vi "BGK Data Acquisition Loop - FCXF.vi"(7 "Period (s)":dbl=600.0 caption="采样周期 (s)" format="%#_13g", 8 "error in (no error)":errorcluster caption="错误输入（无错误）", 11 "Message Queues":T1 caption="消息队列") -> (0 "error out":errorcluster caption="错误输出")   [LabVIEW 2015]
uses:
  Support VIs/Message Queue/All Real-Time Message Queues.ctl
  Support VIs/Message Queue/Message Cluster.ctl
  <vilib>/Platform/TimedLoop/XDataNode/timing_clust.ctl
  <vilib>/Platform/TimedLoop/XDataNode/nitl_modes.ctl
  <vilib>/Platform/TimedLoop/XDataNode/wakeup.ctl
  <vilib>/Instr/_visa.llb/VISA Configure Serial Port (Instr).vi
  Globals/Global - Monitoring Variables.vi
  <vilib>/Platform/TimedLoop/XDataNode/loadnilvce.vi
  Globals/Global - All RT Loop Stop.vi
  <vilib>/Platform/TimedLoop/XDataNode/XDataNode.xnode
  <vilib>/Platform/TimedLoop/XDataNode/XDNodeRunTimeDep.lvlib
  Support VIs/Message Queue/Message Queue.lvlib
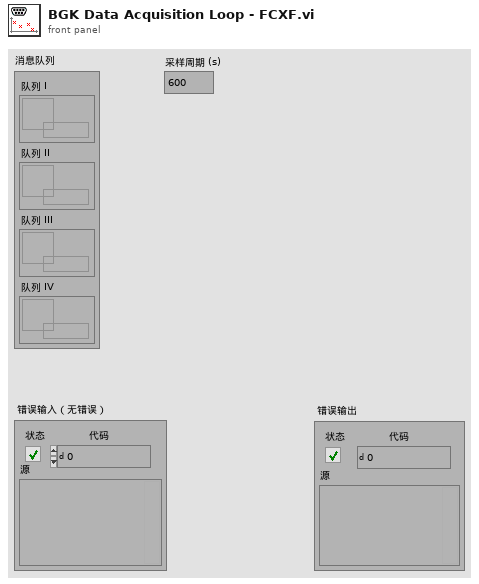
[diagram p1: front panel]
types:
  T1 = typedef "Message Queue.lvlib/All Real-Time Message Queues.ctl" = cluster{"Queue I":refnum<queue>, "Queue II":refnum<queue>, "Queue III":refnum<queue>, "Queue IV":refnum<queue>}
  T2 = typedef "XDNodeRunTimeDep.lvlib/timing_clust.ctl" = cluster{"Expected End [f-1]":u64, "Actual End [f-1]":u64, "Finished Late? [f-1]":bool, "Expected End [i-1]":u64, "Actual End [i-1]":u64, "Finished Late? [i-1]":bool, "Expected Start [i]":u64, "Actual Start [i]":u64, "Expected Start [f]":u64, "Actual Start [f]":u64, "Source Name":string, "Structure Name":string, "Period":i64, "Deadline":i64, "Offset":i64, "Start":i64, "Priority":i32, "Timeout":i32, "Mode":T3, "Wakeup Reason":T4, "Error":errorcluster, "Source Type":string, "Secondary Source Type":string, "Global End Time":u64, "Global Start Time":u64, "Frame Duration":u64, "Iteration Duration":u64, "Assigned CPU":i32, "I/O Scan Engine Mode":u32}
  T3 = typedef "XDNodeRunTimeDep.lvlib/nitl_modes.ctl" = enum32{"No Change", "Process missed periods, maintain original phase", "Discard missed periods, maintain original phase", "Process missed periods, ignore original phase", "Discard missed periods, ignore original phase"}
  T4 = typedef "XDNodeRunTimeDep.lvlib/wakeup.ctl" = enum32{"Normal", "Aborted", "Asynchronous wakeup", "Timing source error", "Timed loop error", "Timeout"}
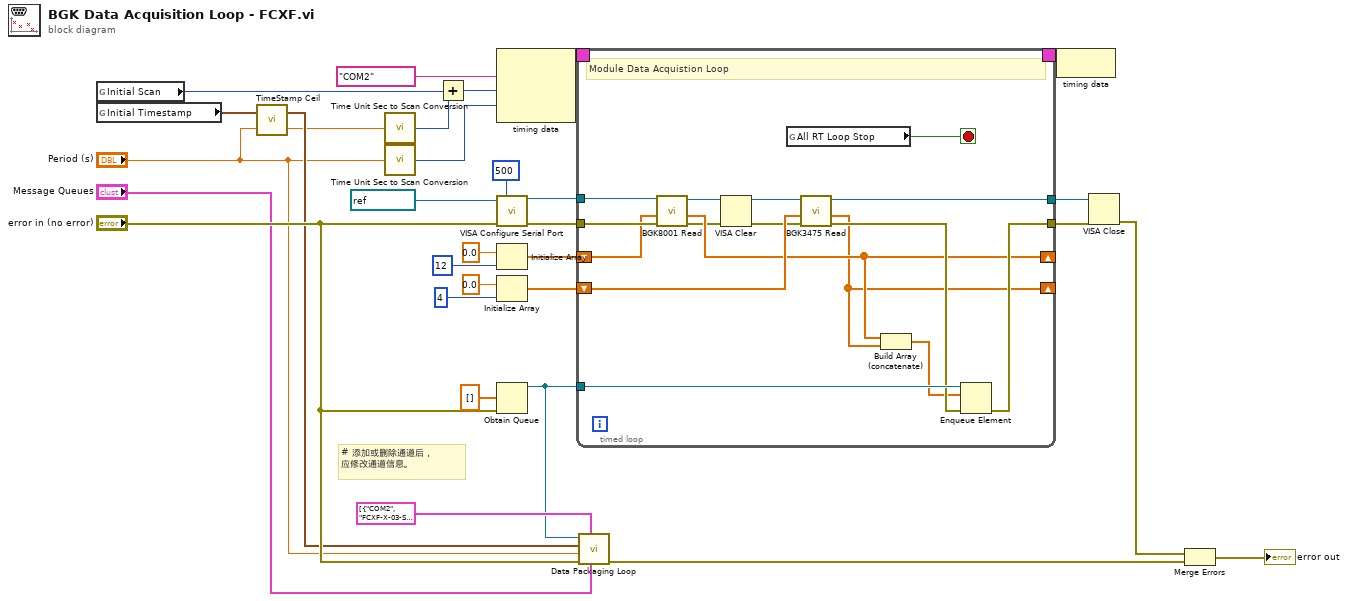
[diagram p0: block diagram]
diagram:
  # "# 添加或删除通道后，\n应修改通道信息。"
  n1 = global read "Global - Monitoring Variables.vi" "Initial Scan"() -> (w17:i64)
  n2 = global read "Global - Monitoring Variables.vi" "Initial Timestamp"() -> (w18:timestamp)
  n3 = call "TimeStamp Ceil.vi"("base (s)"="Period (s)", "timestamp input"=w18) -> ("time diff (s)"=w1:dbl, "timestamp output"=w10:timestamp)
  n4 = call "Time Unit Sec to Scan Conversion.vi"("time duration (s)"=w1) -> ("time duration (scan)"=w16:i64)
  n5 = call "Time Unit Sec to Scan Conversion.vi"("time duration (s)"="Period (s)") -> ("time duration (scan)"=w14:i64)
  n6 = Add(x=w17, y=w16) -> (x+y=w15:i64)
  n7 = node-c288("COM2" ("Structure Name"), w15, w14) -> (w30:T2)
  n8 = call-poly "VISA Configure Serial Port"("VISA resource name"=refnum<visa-resource-name> "COM2", "timeout (10sec)"=u32 500, "error in (no error)"="error in (no error)") -> ("VISA resource name out"=w23:refnum<visa-resource-name>, "error out"=w27:errorcluster)  [unwired: 11 in]
  n9 = Initialize Array(0.0 ("元素"), 12 ("维数大小")) -> (w7:dbl[])
  n10 = Initialize Array(0.0 ("元素"), 4 ("维数大小")) -> (w3:dbl[])
  n11 = Obtain Queue(element data type=dbl[] [] ("数据类型"), error in (no error)="error in (no error)") -> (queue out=w11:refnum<queue>)  [unwired: 3 in, 2 out]
  n12 = timed-loop {
    timing: w30 -> [_]
    timing-out: [_] -> w29
    tunnel: w11 -> [w46]
    tunnel: w27 -> [w39]
    tunnel: [w45] -> w25
    tunnel: [w43] -> w26
    tunnel: w23 -> [w40]
    shift-right: [w36] -> _
    shift-left: w7 -> [w38]
    shift-right: [w35] -> _
    shift-left: w3 -> [w37]
    stop <- w47 stop-if-true
    # "Module Data Acquistion Loop"
    n13 = call "BGK8001 Read.vi"("error in (no error)"=w39, "Last Data Array"=w38, "VISA Ref Input"=w40) -> ("error out"=w33:errorcluster, "New Data Array"=w36:dbl[], "VISA Ref Output"=w44:refnum<visa-resource-name>)  [unwired: 6 in]
    n14 = VISA Clear(VISA resource name=w44, error in (no error)=w33) -> (VISA resource name out=w34:refnum<visa-resource-name>, error out=w32:errorcluster)
    n15 = global read "Global - All RT Loop Stop.vi" "All RT Loop Stop"() -> (w47:bool)
    n16 = call "BGK3475 Read.vi"("error in (no error)"=w32, "Last Data Array"=w37, "VISA Ref Input"=w34) -> ("error out"=w42:errorcluster, "New Data Array"=w35:dbl[], "VISA Ref Output"=w43:refnum<visa-resource-name>)  [unwired: 6 in]
    n17 = Build Array (concatenate)(w36, w35) -> (w41:dbl[])
    n18 = Enqueue Element(queue=w46, element=w41, error in (no error)=w42) -> (error out=w45:errorcluster)  [unwired: 1 in, 2 out]
  }
  n19 = call "Data Packaging Loop.vi"("Message Queues"="Message Queues", "channel info array"=cluster{"Module":string, "Channel":string}[] [{"Module"="COM2", "Channel"="FCXF-X-03-S07"}, {"Module"="COM2", "Channel"="FCXF-X-03-T07"}, {"Module"="COM2", "Channel"="FCXF-X-03-S08"}, {"Module"="COM2", "Channel"="FCXF-X-03-T08"}, {"Module"="COM2", "Channel"="FCXF-X-03-S09"}, {"Module"="COM2", "Channel"="FCXF-X-03-T09"}, {"Module"="COM2", "Channel"="FCXF-X-03-S10"}, {"Module"="COM2", "Channel"="FCXF-X-03-T10"}, {"Module"="COM2", "Channel"="FCXF-X-01-D02"}, {"Module"="COM2", "Channel"="FCXF-X-01-T01"}, {"Module"="COM2", "Channel"="FCXF-X-05-D01"}, {"Module"="COM2", "Channel"="FCXF-X-05-T01"}, {"Module"="COM2", "Channel"="FCXF-X-01-D01"}, {"Module"="COM2", "Channel"="FCXF-X-02-D01"}, {"Module"="COM2", "Channel"="FCXL-X-03-D01"}, {"Module"="COM2", "Channel"="FCXF-X-04-D01"}], "error in (no error)"="error in (no error)", "sampling period (s)"="Period (s)", "timestamp"=w10, "data queue"=w11) -> ("error out"=w19:errorcluster)  [unwired: 5 in]
  n20 = node-c288(w29) -> ()
  n21 = VISA Close(VISA resource name=w26, error in (no error)=w25) -> (error out=w24:errorcluster)
  n22 = Merge Errors(w24, w19) -> (→"error out":errorcluster)
